vi "Main.vi"() -> ()   [LabVIEW 2021]
doc: "The myRIO Project template acquires acceleration data from the onboard accelerometer and displays the changes of acceleration values in a waveform chart."
uses:
  <vilib>/myRIO/Instrument Drivers/Onboard IO/AI/typedefs/AI Reference.ctl
  <vilib>/myRIO/Common/Instrument Driver Framework/Utilities/typedefs/myRIO Generic Hardware Reference.ctl
  <vilib>/myRIO/Common/Instrument Driver Framework/Utilities/typedefs/Hardware Version Enum.ctl
  <vilib>/myRIO/Common/Instrument Driver Framework/Utilities/typedefs/myRIO v1.0 Reference.ctl
  <vilib>/myRIO/Common/Instrument Driver Framework/Utilities/typedefs/Generic FPGA Reference.ctl
  <vilib>/myRIO/Common/Instrument Driver Framework/myRIO v1.0/AI/typedefs/AI Channels List.ctl
  <vilib>/myRIO/Common/Instrument Driver Framework/myRIO v1.0/AI/typedefs/AI Channels Enum.ctl
  <vilib>/myRIO/Common/Instrument Driver Framework/Utilities/typedefs/Analog Scaling Constants List.ctl
  <vilib>/myRIO/Common/Instrument Driver Framework/Utilities/typedefs/Analog Scaling Constants.ctl
  <vilib>/userDefined/High Color/nirio_resource_hc.ctl
  <vilib>/myRIO/Instrument Drivers/Onboard IO/DIO/typedefs/DIO Reference.ctl
  <vilib>/myRIO/Common/Instrument Driver Framework/myRIO v1.0/DIO/typedefs/DIO Channels List.ctl
  <vilib>/myRIO/Common/Instrument Driver Framework/myRIO v1.0/DIO/typedefs/DIO Channels Enum.ctl
  <vilib>/myRIO/Instrument Drivers/Onboard IO/PWM/typedefs/PWM Reference.ctl
  <vilib>/myRIO/Common/Instrument Driver Framework/myRIO v1.0/PWM/typedefs/PWM Channels Enum.ctl
  <vilib>/myRIO/Instrument Drivers/Onboard IO/PWM/typedefs/PWM Configuration.ctl
  <vilib>/myRIO/Common/Instrument Driver Framework/Utilities/vis/Is FPGA Ref Available.vi
  <vilib>/myRIO/Common/Instrument Driver Framework/myRIO v1.0/AI/vis/myRIO v1.1 Open AI.vi
  <vilib>/myRIO/Instrument Drivers/Onboard IO/AI/vis/Read.vi
  <vilib>/myRIO/Common/Instrument Driver Framework/myRIO v1.0/DIO/vis/myRIO v1.1 Open DIO.vi
  <vilib>/myRIO/Instrument Drivers/Onboard IO/DIO/vis/Write.vi
  <vilib>/myRIO/Common/Instrument Driver Framework/myRIO v1.0/PWM/vis/myRIO v1.1 Open PWM.vi
  <vilib>/myRIO/Instrument Drivers/Onboard IO/PWM/vis/Set Duty Cycle and Frequency.vi
  <vilib>/myRIO/Instrument Drivers/Onboard IO/DIO/vis/Read.vi
  <vilib>/myRIO/Common/Instrument Driver Framework/Utilities/vis/Validate Channels.vi
  <vilib>/myRIO/Common/Instrument Driver Framework/myRIO v1.0/AI/vis/myRIO v1.0 Reserve AI.vi
  <vilib>/myRIO/Common/Instrument Driver Framework/myRIO v1.0/DIO/vis/myRIO v1.0 Reserve DIO.vi
  <vilib>/myRIO/Common/Instrument Driver Framework/myRIO v1.0/PWM/vis/myRIO v1.0 Reserve PWM.vi
  <vilib>/myRIO/Common/Instrument Driver Framework/myRIO v1.0/UART/vis/myRIO v1.0 Close UART.vi
  <vilib>/myRIO/Common/Instrument Driver Framework/myRIO v1.0/AI/vis/myRIO v1.0 Build MUX Configuration AI.vi
  <vilib>/myRIO/Common/Instrument Driver Framework/myRIO v1.0/Resource Manager/vis/myRIO v1.0 Reserve Channel List.vi
  <vilib>/myRIO/Common/Instrument Driver Framework/myRIO v1.0/DIO/vis/myRIO v1.0 Build MUX Configuration DIO.vi
  <vilib>/myRIO/Common/Instrument Driver Framework/myRIO v1.0/PWM/vis/myRIO v1.0 Build MUX Configuration PWM.vi
  <vilib>/myRIO/Common/Instrument Driver Framework/myRIO v1.0/Resource Manager/vis/myRIO v1.0 Reserve Channel.vi
  <vilib>/myRIO/Common/Instrument Driver Framework/myRIO v1.0/Resource Manager/vis/myRIO v1.0 Unreserve Channel.vi
  <vilib>/myRIO/Common/Instrument Driver Framework/myRIO v1.0/Resource Manager/vis/myRIO v1.0 Create Configuration List.vi
  <vilib>/myRIO/Common/Instrument Driver Framework/myRIO v1.0/Resource Manager/vis/myRIO v1.0 Build Mutex Name.vi
  <vilib>/Utility/VariantDataType/GetNumericInfo.vi
  <vilib>/Utility/error.llb/Error Cluster From Error Code.vi
  <vilib>/myRIO/Common/Instrument Driver Framework/myRIO v1.0/myRIO v1.1 Open.vi
  <vilib>/myRIO/Common/Instrument Driver Framework/Utilities/vis/IO Manager.vi
  <vilib>/myRIO/Common/Instrument Driver Framework/Utilities/vis/Configuration Manager.vi
  <vilib>/myRIO/Common/Instrument Driver Framework/myRIO v1.0/Resource Manager/vis/myRIO v1.0 Configure IO.vi
  <vilib>/myRIO/Common/Instrument Driver Framework/myRIO v1.0/myRIO v1.0 Close.vi
  <vilib>/myRIO/Common/Instrument Driver Framework/myRIO v1.0/PWM/vis/myRIO v1.0 Write PWM.vi
  <vilib>/myRIO/Common/Instrument Driver Framework/myRIO v1.0/DIO/vis/myRIO v1.0 Write DIO.vi
  <vilib>/myRIO/Common/Instrument Driver Framework/myRIO v1.0/AI/vis/myRIO v1.0 Get Scaling Constants AI.vi
  <vilib>/myRIO/Common/Instrument Driver Framework/myRIO v1.0/AI/vis/myRIO v1.0 Read AI.vi
  <vilib>/myRIO/Common/Instrument Driver Framework/myRIO v1.0/DIO/vis/myRIO v1.0 Read DIO.vi
  <vilib>/addons/control/pid/pid.llb/PID (DBL).vi
  <vilib>/myRIO/Common/Instrument Driver Framework/Utilities/vis/FPGA Ref Manager.vi
  <vilib>/myRIO/Common/Instrument Driver Framework/myRIO v1.0/myRIO v1.0 Reset FPGA.vi
  <vilib>/myRIO/Common/Instrument Driver Framework/myRIO v1.0/IRQ/vis/myRIO v1.0 IRQ Info FGV.vi
  <vilib>/myRIO/Common/Instrument Driver Framework/myRIO v1.0/IRQ/vis/myRIO v1.0 Timer IRQ Info FGV.vi
  <vilib>/myRIO/Common/Instrument Driver Framework/myRIO v1.0/IRQ/vis/myRIO v1.0 ISR Agent.vi
  <vilib>/myRIO/Instrument Drivers/Utilities/vis/Reset Index.vi
  <vilib>/myRIO/Common/Instrument Driver Framework/myRIO v1.0/Resource Manager/vis/myRIO v1.0 Block Write Resource Manager.vi
  <vilib>/myRIO/Express VI/Onboard IO/PWM/PWM Express VI.xnode
  <vilib>/myRIO/Instrument Drivers/Onboard IO/PWM/vis/myRIO PWM Open.xnode
  <vilib>/myRIO/Express VI/Onboard IO/DO/DO Express VI.xnode
  <vilib>/myRIO/Instrument Drivers/Onboard IO/DIO/vis/myRIO DIO Open.xnode
  <vilib>/myRIO/Express VI/Onboard Devices/LED/LED Express VI.xnode
  <vilib>/myRIO/Express VI/Onboard IO/AI/AI Express VI.xnode
  <vilib>/myRIO/Instrument Drivers/Onboard IO/AI/vis/myRIO AI Open.xnode
  <vilib>/myRIO/Express VI/Onboard IO/DI/DI Express VI.xnode
  <vilib>/myRIO/Instrument Drivers/Utilities/Utilities.lvlib
  <vilib>/myRIO/Instrument Drivers/Onboard IO/PWM/PWM.lvlib
  <vilib>/myRIO/Instrument Drivers/Onboard IO/DIO/DIO.lvlib
  <vilib>/myRIO/Instrument Drivers/Onboard IO/AI/AI.lvlib
  <vilib>/addons/control/pid/NI_PID_pid.lvlib
panel:
  in  "reinitialize? (F)":bool=TRUE
  out "Count":dbl=50.0
  in  "Sensor Threshold":dbl(slide)=3.5112359550561796 scale=0.0..5.0
  out "Waveform Chart":cluster{"Pick Angle":dbl, "Angle":dbl}(graph)={"Pick Angle"=150.0, "Angle"=119.60447994000002}
  in  "Start":bool
  in  "PID gains":T1={"proportional gain (Kc)"=0.008, "integral time (Ti, min)"=1000.0, "derivative time (Td, min)"=0.5} {"derivative time (Td, min)" format="%.3f"; "integral time (Ti, min)" format="%.3f"; "proportional gain (Kc)" format="%.3f"}
  out "LED Sensor":dbl=1.56249984
  out "Angle Stack":T2={"Stack"=[116.96776146, 117.04100364000001, 119.60447994000002, 116.74803492000001, 116.74803492000001, 116.74803492000001, 116.8212771, 116.8212771, 116.89451928000001, 116.96776146], "Stack Pointer"=3.0, "Stack Size"=10.0}
  in  "State":T3(ring)=enum."Sensor-Place"
  in  "Wait Times (ms)":cluster{"Pick Time":dbl, "Sensor Time":dbl}={"Pick Time"=50.0, "Sensor Time"=2000.0}
  in  "Automatic Control Angles (deg)":T4={"Pick Angle"=90.0, "Sensor Angle"=122.0, "Place Angle"=150.0, "Threshold"=5.0}
  in  "Stop Button":bool
  # "Settings For Automatic Control"
  # "Internal"
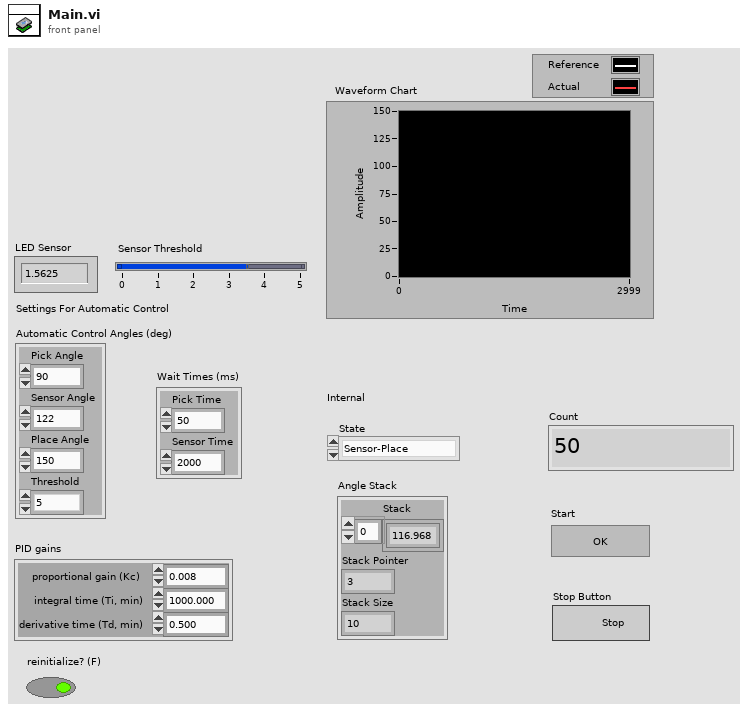
[diagram p1: front panel]
types:
  T1 = cluster{"proportional gain (Kc)":dbl, "integral time (Ti, min)":dbl, "derivative time (Td, min)":dbl}
  T2 = cluster{"Stack":dbl[], "Stack Pointer":dbl, "Stack Size":dbl}
  T3 = enum16{"Manual", "Pick", "Pick-Sensor", "Sensor", "Sensor-Place", "Place", "Place-Pick"}
  T4 = cluster{"Pick Angle":dbl, "Sensor Angle":dbl, "Place Angle":dbl, "Threshold":dbl}
  T5 = typedef "AI.lvlib/AI Reference.ctl" = cluster{"myRIO Reference":T6, "AI Channels List":T10, "AI Scaling Constants List":T12}
  T6 = typedef "myRIO Generic Hardware Reference.ctl" = cluster{"myRIO Model":T7, "myRIO Hardware Reference":T8}
  T7 = typedef "Hardware Version Enum.ctl" = enum16{"Unknown", "myRIO-1900", "myRIO-1950", "roboRIO", "NI ELVIS RIO CM", "ELVIS III"}
  T8 = typedef "myRIO v1.0 Reference.ctl" = cluster{"Generic FPGA Reference":T9, "Allow multiple opens":bool}
  T9 = typedef "Generic FPGA Reference.ctl" = refnum<k20>
  T10 = typedef "AI Channels List.ctl" = T11[]
  T11 = typedef "AI Channels Enum.ctl" = enum16{"Not Connected", "AudioIn/Left", "AudioIn/Right", "C/AI0", "C/AI1", "A/AI0", "A/AI1", "A/AI2", "A/AI3", "A/AI4", "A/AI5", "A/AI6", "A/AI7", "B/AI0", "B/AI1", "B/AI2", "B/AI3", "B/AI4", "B/AI5", "B/AI6", "B/AI7", "AI/AI0", "AI/AI1", "AI/AI2", "AI/AI3", "A/AI0 (DIFF)", "A/AI1 (DIFF)", "A/AI2 (DIFF)", "A/AI3 (DIFF)", "B/AI0 (DIFF)", "B/AI1 (DIFF)", "B/AI2 (DIFF)", "B/AI3 (DIFF)"}
  T12 = typedef "Analog Scaling Constants List.ctl" = T13[]
  T13 = typedef "Analog Scaling Constants.ctl" = cluster{"LSB Weight (Volts)":dbl, "Offset (Volts)":dbl, "Signed?":bool}
  T14 = typedef "nirio_resource_hc.ctl" = tag
  T15 = typedef "DIO.lvlib/DIO Reference.ctl" = cluster{"myRIO Reference":T6, "DIO Channels List":T16}
  T16 = typedef "DIO Channels List.ctl" = T17[]
  T17 = typedef "DIO Channels Enum.ctl" = enum16{"Not Connected", "C/DIO0", "C/DIO1", "C/DIO2", "C/DIO3", "C/DIO4", "C/DIO5", "C/DIO6", "C/DIO7", "A/DIO0", "A/DIO1", "A/DIO2", "A/DIO3", "A/DIO4", "A/DIO5", "A/DIO6", "A/DIO7", "A/DIO8", "A/DIO9", "A/DIO10", "A/DIO11", "A/DIO12", "A/DIO13", "A/DIO14", "A/DIO15", "A/DIO16", "A/DIO17", "A/DIO18", "A/DIO19", "B/DIO0", "B/DIO1", "B/DIO2", "B/DIO3", "B/DIO4", "B/DIO5", "B/DIO6", "B/DIO7", "B/DIO8", "B/DIO9", "B/DIO10", "B/DIO11", "B/DIO12", "B/DIO13", "B/DIO14", "B/DIO15", "B/DIO16", "B/DIO17", "B/DIO18", "B/DIO19", "LED0", "LED1", "LED2", "LED3", "Button0", "DIO/DIO0", "DIO/DIO1", "DIO/DIO2", "DIO/DIO3", "DIO/DIO4", "DIO/DIO5", "DIO/DIO6", "DIO/DIO7", "DIO/DIO8", "DIO/DIO9", "SPI/CS0", "SPI/CS1", "SPI/CS2", "SPI/CS3", "LED RADIO (Green)", "LED RADIO (Red)", "LED COMM (Green)", "LED COMM (Red)", "LED MODE (Green)", "LED MODE (Red)"}
  T18 = typedef "PWM.lvlib/PWM Reference.ctl" = cluster{"myRIO Reference":T6, "PWM Channels Enum":T19, "PWM Configuration":T20}
  T19 = typedef "PWM Channels Enum.ctl" = enum16{"Not Connected", "C/PWM0", "C/PWM1", "A/PWM0", "A/PWM1", "A/PWM2", "A/PWM3", "A/PWM4", "A/PWM5", "A/PWM6", "A/PWM7", "A/PWM8", "A/PWM9", "A/PWM10", "A/PWM11", "A/PWM12", "A/PWM13", "A/PWM14", "A/PWM15", "A/PWM16", "A/PWM17", "A/PWM18", "A/PWM19", "B/PWM0", "B/PWM1", "B/PWM2", "B/PWM3", "B/PWM4", "B/PWM5", "B/PWM6", "B/PWM7", "B/PWM8", "B/PWM9", "B/PWM10", "B/PWM11", "B/PWM12", "B/PWM13", "B/PWM14", "B/PWM15", "B/PWM16", "B/PWM17", "B/PWM18", "B/PWM19", "PWM/PWM0", "PWM/PWM1", "PWM/PWM2", "PWM/PWM3", "PWM/PWM4", "PWM/PWM5", "PWM/PWM6", "PWM/PWM7", "PWM/PWM8", "PWM/PWM9"}
  T20 = typedef "PWM.lvlib/PWM Configuration.ctl" = cluster{"Frequency":dbl, "Duty Cycle":dbl}
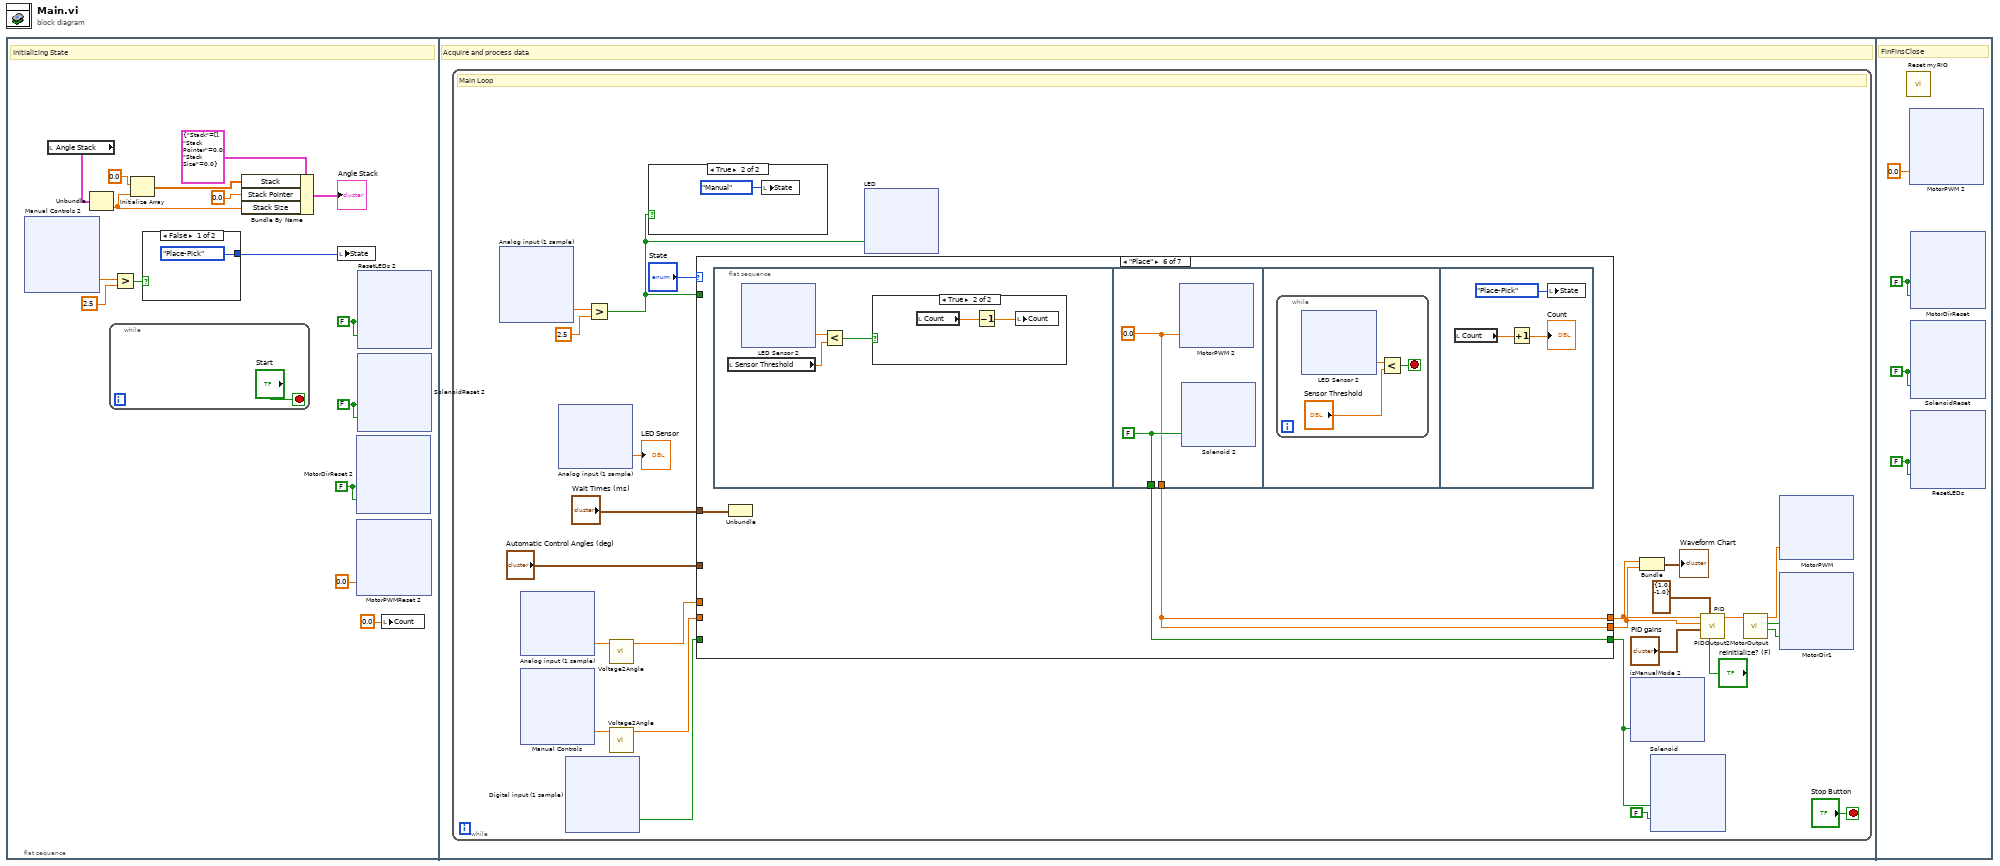
[diagram p0: block diagram]
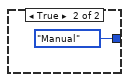
[diagram p2: hidden frame]
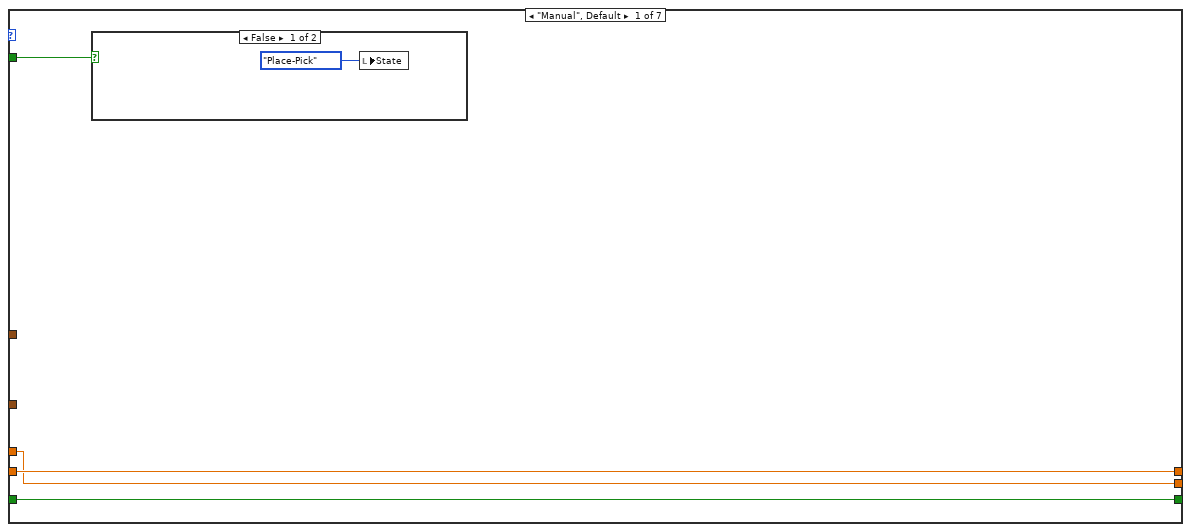
[diagram p4: hidden frame]
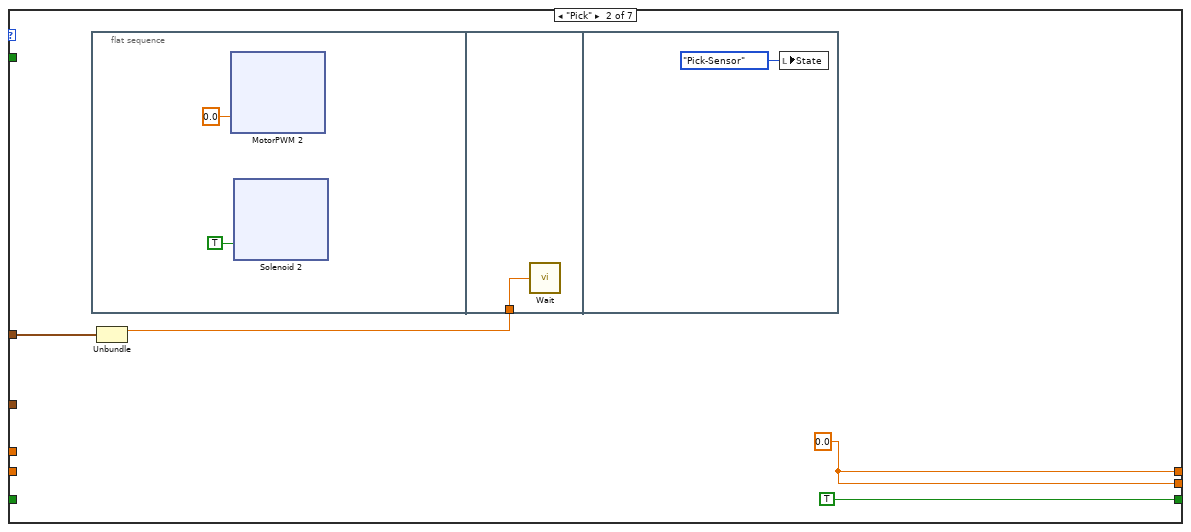
[diagram p6: hidden frame]
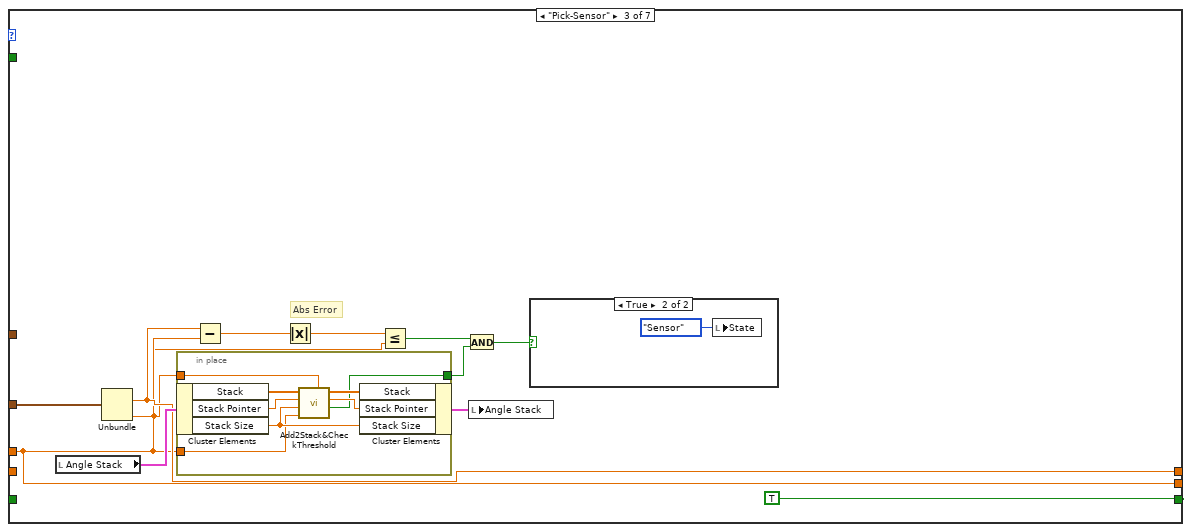
[diagram p7: hidden frame]
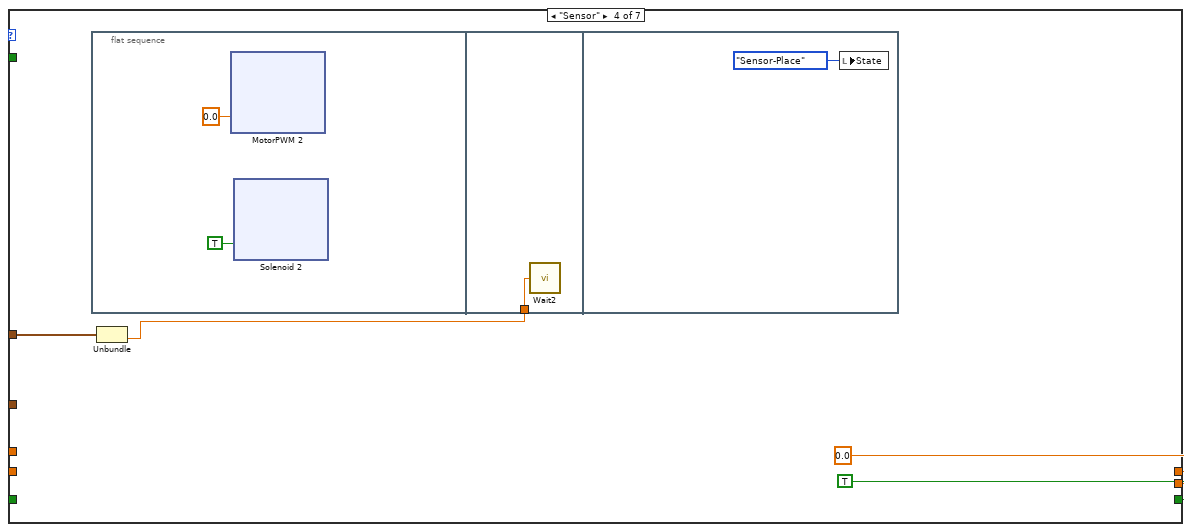
[diagram p9: hidden frame]
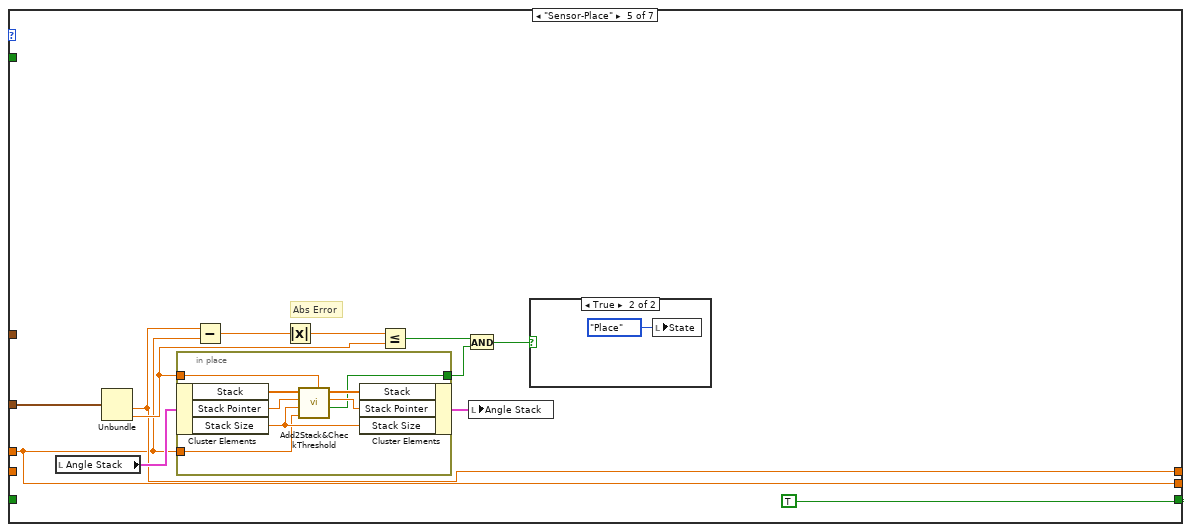
[diagram p10: hidden frame]
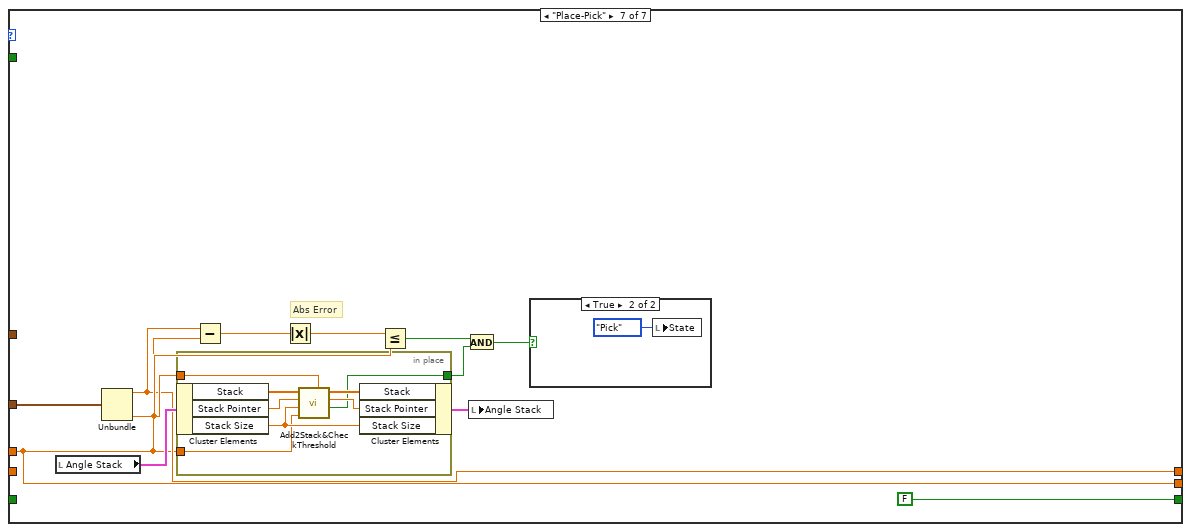
[diagram p13: hidden frame]
diagram:
  n1 = flat-sequence {
    frame #0 {
      w5 = FALSE ("LED0")
      w6 = FALSE ("Solenoid1 (A/DIO2 (Pin 15))")
      w7 = FALSE
      # "Initializing State"
      n2 = xnode "Manual Controls 2"() -> ("isManualMode (A/AI3 (Pin 9))"=w3:dbl)  [unwired: 1 in, 1 out]
      n3 = local read "Angle Stack"() -> (w13:T2)
      n4 = Unbundle(w13) -> ("Stack Size"=w9:dbl)  [unwired: 2 out]
      n5 = while {
        stop <- "Start" stop-if-true
      }
      n6 = Greater?(x=w3, y=2.5) -> (0:w1:bool)
      n7 = Initialize Array(0.0 ("element"), w9) -> (w10:dbl[])
      n8 = case shown="False" w1 {
        tunnel: [T3."Place-Pick" ("State") T3."Manual" ("State")] -> w16
        frame False {
        }
        frame True {
        }
      }
      n9 = Bundle By Name(cluster=T2 {"Stack"=[], "Stack Pointer"=0.0, "Stack Size"=0.0} ("Angle Stack"), "Stack"=w10, "Stack Pointer"=0.0, "Stack Size"=w9) -> (→"Angle Stack":T2)
      n10 = local write "State"(w16) -> ()
      n11 = xnode "MotorDirReset 2"("MotorDir1 (A/DIO0 (Pin 11))"=w7, "MotorDir2 (A/DIO1 (Pin 13))"=w7) -> ()  [unwired: 1 in, 1 out]
      n12 = xnode "MotorPWMReset 2"("Duty Cycle"=0.0) -> ()  [unwired: 1 in, 1 out]
      n13 = xnode "ResetLEDs 2"("LED0"=w5, "LED1"=w5) -> ()  [unwired: 1 in, 1 out]
      n14 = xnode "SolenoidReset 2"("Solenoid1 (A/DIO2 (Pin 15))"=w6, "Solenoid2 (A/DIO3 (Pin 17))"=w6) -> ()  [unwired: 1 in, 1 out]
      n15 = local write "Count"(0.0 ("Count")) -> ()
    }
    frame #1 {
      # "Acquire and process data"
      n16 = while {
        stop <- "Stop Button" stop-if-true
        # "Main Loop"
        n17 = xnode "Analog input (1 sample)"() -> ("isManualMode (A/AI3 (Pin 9))"=w203:dbl)  [unwired: 1 in, 1 out]
        n18 = xnode "Analog input (1 sample)"() -> ("Angle (A/AI0 (Pin 3))"=w223:dbl)  [unwired: 1 in, 1 out]
        n19 = xnode "Manual Controls"() -> ("Angle (A/AI2 (Pin 7))"=w206:dbl)  [unwired: 1 in, 1 out]
        n20 = xnode "Analog input (1 sample)"() -> ("LED Sensor (A/AI1 (Pin 5))"=→"LED Sensor":dbl)  [unwired: 1 in, 1 out]
        n21 = xnode "Digital input (1 sample)"() -> ("Magnet (A/DIO5 (Pin 21))"=w205:bool)  [unwired: 1 in, 1 out]
        n22 = Greater?(x=w203, y=2.5) -> (0:w201:bool)
        n23 = call "Voltage2Angle.vi"("Voltage"=w223) -> ("Angle"=w209:dbl)  [unwired: 10 in]
        n24 = call "Voltage2Angle.vi"("Voltage"=w206) -> ("Angle"=w213:dbl)  [unwired: 10 in]
        n25 = case shown="True" w201 {
          frame False {
          }
          frame True {
            n26 = local write "State"(T3."Manual" ("State")) -> ()
          }
        }
        n27 = case shown="\"Place\"" "State" {
          tunnel: "Wait Times (ms)" -> [_ w378 _ w477 _ w575 _]
          tunnel: "Automatic Control Angles (deg)" -> [_ _ w462 _ w555 _ w735]
          tunnel: w209 -> [w372 _ w458 _ w552 _ w733]
          tunnel: w213 -> [w373 _ _ _ _ _ _]
          tunnel: w205 -> [w371 _ _ _ _ _ _]
          tunnel: [w373 w375 w459 w474 w554 w574 w734] -> w211
          tunnel: [w372 w375 w458 w474 w552 w574 w733] -> w210
          tunnel: [w371 TRUE ("Solenoid") TRUE ("Solenoid") TRUE ("Solenoid") TRUE ("Solenoid") w573 FALSE ("Solenoid")] -> w208
          tunnel: w201 -> [w370 _ _ _ _ _ _]
          frame "Manual", Default {
            n28 = case shown="False" w370 {
              frame False {
                n29 = local write "State"(T3."Place-Pick" ("State")) -> ()
              }
              frame True {
              }
            }
          }
          frame "Pick" {
            w375 = 0.0 ("Pick Angle")
            n30 = flat-sequence {
              tunnel: w377 -> [w451]
              frame #0 {
                n31 = xnode "MotorPWM 2"("Duty Cycle"=0.0) -> ()  [unwired: 1 in, 1 out]
                n32 = xnode "Solenoid 2"("Solenoid1 (A/DIO2 (Pin 15))"=TRUE) -> ()  [unwired: 1 in, 1 out]
              }
              frame #1 {
                n33 = call "Wait"("Count(mSec)"=w451) -> ()  [unwired: 1 out]
              }
              frame #2 {
                n34 = local write "State"(T3."Pick-Sensor" ("State")) -> ()
              }
            }
            n35 = Unbundle(w378) -> ("Pick Time"=w377:dbl)  [unwired: 1 out]
          }
          frame "Pick-Sensor" {
            # "Abs Error"
            n36 = local read "Angle Stack"() -> (w464:T2)
            n37 = Unbundle(w462) -> ("Sensor Angle"=w459:dbl, "Threshold"=w455:dbl)  [unwired: 2 out]
            n38 = in-place {
              in-place-border: w458 -> [w468]
              in-place-border: w455 -> [w467]
              in-place-border: [w466] -> w460
              n39 = in-place-cluster #1(w464) -> ("Stack"=w473:dbl[], "Stack Pointer"=w472:dbl, "Stack Size"=w471:dbl)
              n40 = call "Add2Stack&CheckThreshold.vi"("Stack In"=w473, "Stack Pointer  In"=w472, "Stack Size"=w471, "Angle"=w468, "Threshold"=w467) -> ("Stack Out"=w469:dbl[], "Stack Pointer Out"=w470:dbl, "Threshold Reached"=w466:bool)  [unwired: 2 in]
              n41 = in-place-cluster #1("Stack"=w469, "Stack Pointer"=w470, "Stack Size"=w471) -> (w463:T2)
            }
            n42 = Subtract(x=w459, y=w458) -> (x-y=w457:dbl)
            n43 = Absolute Value(x=w457) -> (abs(x)=w456:dbl)
            n44 = Less Or Equal?(x=w456, y=w455) -> (x <= y?=w454:bool)
            n45 = And(x=w454, y=w460) -> (x .and. y?=w461:bool)
            n46 = local write "Angle Stack"(w463) -> ()
            n47 = case shown="True" w461 {
              frame False {
              }
              frame True {
                n48 = local write "State"(T3."Sensor" ("State")) -> ()
              }
            }
          }
          frame "Sensor" {
            w474 = 0.0 ("Pick Angle")
            n49 = flat-sequence {
              tunnel: w476 -> [w550]
              frame #0 {
                n50 = xnode "MotorPWM 2"("Duty Cycle"=0.0) -> ()  [unwired: 1 in, 1 out]
                n51 = xnode "Solenoid 2"("Solenoid1 (A/DIO2 (Pin 15))"=TRUE) -> ()  [unwired: 1 in, 1 out]
              }
              frame #1 {
                n52 = call "Wait2"("Count(mSec)"=w550) -> ()  [unwired: 1 out]
              }
              frame #2 {
                n53 = local write "State"(T3."Sensor-Place" ("State")) -> ()
              }
            }
            n54 = Unbundle(w477) -> ("Sensor Time"=w476:dbl)  [unwired: 1 out]
          }
          frame "Sensor-Place" {
            # "Abs Error"
            n55 = local read "Angle Stack"() -> (w563:T2)
            n56 = Unbundle(w555) -> ("Place Angle"=w554:dbl, "Threshold"=w557:dbl)  [unwired: 2 out]
            n57 = in-place {
              in-place-border: w552 -> [w567]
              in-place-border: w557 -> [w566]
              in-place-border: [w565] -> w560
              n58 = in-place-cluster #2(w563) -> ("Stack"=w572:dbl[], "Stack Pointer"=w571:dbl, "Stack Size"=w570:dbl)
              n59 = call "Add2Stack&CheckThreshold.vi"("Stack In"=w572, "Stack Pointer  In"=w571, "Stack Size"=w570, "Angle"=w567, "Threshold"=w566) -> ("Stack Out"=w568:dbl[], "Stack Pointer Out"=w569:dbl, "Threshold Reached"=w565:bool)  [unwired: 2 in]
              n60 = in-place-cluster #2("Stack"=w568, "Stack Pointer"=w569, "Stack Size"=w570) -> (w562:T2)
            }
            n61 = Subtract(x=w554, y=w552) -> (x-y=w559:dbl)
            n62 = Absolute Value(x=w559) -> (abs(x)=w558:dbl)
            n63 = Less Or Equal?(x=w558, y=w557) -> (x <= y?=w556:bool)
            n64 = And(x=w556, y=w560) -> (x .and. y?=w561:bool)
            n65 = local write "Angle Stack"(w562) -> ()
            n66 = case shown="True" w561 {
              frame False {
              }
              frame True {
                n67 = local write "State"(T3."Place" ("State")) -> ()
              }
            }
          }
          frame "Place" {
            n68 = flat-sequence {
              tunnel: [w618] -> w574
              tunnel: [w619] -> w573
              frame #0 {
                n69 = local read "Sensor Threshold"() -> (w577:dbl)
                n70 = xnode "LED Sensor 2"() -> ("LED Sensor (A/AI1 (Pin 5))"=w576:dbl)  [unwired: 1 in, 1 out]
                n71 = Less?(x=w576, y=w577) -> (x < y?=w578:bool)
                n72 = case shown="True" w578 {
                  frame False {
                  }
                  frame True {
                    n73 = local read "Count"() -> (w617:dbl)
                    n74 = Decrement(x=w617) -> (x-1=w616:dbl)
                    n75 = local write "Count"(w616) -> ()
                  }
                }
              }
              frame #1 {
                w618 = 0.0
                w619 = FALSE
                n76 = xnode "MotorPWM 2"("Duty Cycle"=w618) -> ()  [unwired: 1 in, 1 out]
                n77 = xnode "Solenoid 2"("Solenoid1 (A/DIO2 (Pin 15))"=w619) -> ()  [unwired: 1 in, 1 out]
              }
              frame #2 {
                n78 = while {
                  stop <- w692 stop-if-true
                  n79 = xnode "LED Sensor 2"() -> ("LED Sensor (A/AI1 (Pin 5))"=w691:dbl)  [unwired: 1 in, 1 out]
                  n80 = Less?(x=w691, y="Sensor Threshold") -> (x < y?=w692:bool)
                }
              }
              frame #3 {
                n81 = local read "Count"() -> (w730:dbl)
                n82 = Increment(x=w730) -> (x+1=→"Count":dbl)
                n83 = local write "State"(T3."Place-Pick" ("State")) -> ()
              }
            }
            n84 = Unbundle(w575) -> ()  [unwired: 2 out]
          }
          frame "Place-Pick" {
            # "Abs Error"
            n85 = local read "Angle Stack"() -> (w744:T2)
            n86 = Unbundle(w735) -> ("Pick Angle"=w734:dbl, "Threshold"=w738:dbl)  [unwired: 2 out]
            n87 = in-place {
              in-place-border: w733 -> [w748]
              in-place-border: w738 -> [w747]
              in-place-border: [w746] -> w741
              n88 = in-place-cluster #3(w744) -> ("Stack"=w753:dbl[], "Stack Pointer"=w752:dbl, "Stack Size"=w751:dbl)
              n89 = call "Add2Stack&CheckThreshold.vi"("Stack In"=w753, "Stack Pointer  In"=w752, "Stack Size"=w751, "Angle"=w748, "Threshold"=w747) -> ("Stack Out"=w749:dbl[], "Stack Pointer Out"=w750:dbl, "Threshold Reached"=w746:bool)  [unwired: 2 in]
              n90 = in-place-cluster #3("Stack"=w749, "Stack Pointer"=w750, "Stack Size"=w751) -> (w743:T2)
            }
            n91 = Subtract(x=w734, y=w733) -> (x-y=w740:dbl)
            n92 = Absolute Value(x=w740) -> (abs(x)=w739:dbl)
            n93 = Less Or Equal?(x=w739, y=w738) -> (x <= y?=w737:bool)
            n94 = And(x=w737, y=w741) -> (x .and. y?=w742:bool)
            n95 = local write "Angle Stack"(w743) -> ()
            n96 = case shown="True" w742 {
              frame False {
              }
              frame True {
                n97 = local write "State"(T3."Pick" ("State")) -> ()
              }
            }
          }
        }
        n98 = xnode "LED"("LED0"=w201) -> ()  [unwired: 1 in, 1 out]
        n99 = xnode "isManualMode 2"("LED1"=w208) -> ()  [unwired: 1 in, 1 out]
        n100 = Bundle("Pick Angle"=w211, "Angle"=w210) -> (→"Waveform Chart":cluster{"Pick Angle":dbl, "Angle":dbl})  [unwired: 1 in]
        n101 = xnode "Solenoid"("Solenoid1 (A/DIO2 (Pin 15))"=w208, "Solenoid2 (A/DIO3 (Pin 17))"=FALSE) -> ()  [unwired: 1 in, 1 out]
        n102 = call-poly <vilib>:"PID.vi"("reinitialize? (F)"="reinitialize? (F)", "output range"=cluster{"output high":dbl, "output low":dbl} {"output high"=1.0, "output low"=-1.0}, "PID gains"="PID gains", "process variable"=w210, "setpoint"=w211) -> ("output"=w214:dbl)  [unwired: 5 in, 1 out]
        n103 = call "PIDOutput2MotorOutput.vi"("PID Output"=w214) -> ("Dir2"=w220:bool, "Dir1"=w221:bool, "Duty Cycle"=w222:dbl)  [unwired: 8 in]
        n104 = xnode "MotorPWM"("Duty Cycle"=w222) -> ()  [unwired: 1 in, 1 out]
        n105 = xnode "MotorDir1"("MotorDir1 (A/DIO0 (Pin 11))"=w221, "MotorDir2 (A/DIO1 (Pin 13))"=w220) -> ()  [unwired: 1 in, 1 out]
      }
    }
    frame #2 {
      w970 = FALSE ("LED0")
      w971 = FALSE ("Solenoid1 (A/DIO2 (Pin 15))")
      w972 = FALSE
      # "FinFinsClose"
      n106 = call <vilib>:"Reset myRIO.vi"() -> ()  [unwired: 11 in, 1 out]
      n107 = xnode "MotorPWM 2"("Duty Cycle"=0.0) -> ()  [unwired: 1 in, 1 out]
      n108 = xnode "MotorDirReset"("MotorDir1 (A/DIO0 (Pin 11))"=w972, "MotorDir2 (A/DIO1 (Pin 13))"=w972) -> ()  [unwired: 1 in, 1 out]
      n109 = xnode "SolenoidReset"("Solenoid1 (A/DIO2 (Pin 15))"=w971, "Solenoid2 (A/DIO3 (Pin 17))"=w971) -> ()  [unwired: 1 in, 1 out]
      n110 = xnode "ResetLEDs"("LED0"=w970, "LED1"=w970) -> ()  [unwired: 1 in, 1 out]
    }
  }
